vi "Autonomous Independent.vi"   [LabVIEW 2013]
doc: "This VI is called when autonomous begins, and will automatically be terminated when autonomous ends. You can carry out timed or sensor driven robot movement independently without needing to return to the caller."
uses:
  Robot Global Data.vi
  <vilib>/Rock Robotics/WPI/Counter/WPI_CounterDigitalInputToDigitalSource.vi
types:
  T1 = cluster{"Open Claw?":bool, "Close Claw?":bool, "Minibot Out":bool}
  T2 = typedef "WPI_DigitalInputDevRef.ctl" = cluster{"DevStatus":errorcluster, "DIO Channel":T3, "Digital Module":T4}
  T3 = typedef "FPGA_DIOChannel.ctl" = enum8{"DIO 1", "DIO 2", "DIO 3", "DIO 4", "DIO 5", "DIO 6", "DIO 7", "DIO 8", "DIO 9", "DIO 10", "DIO 11", "DIO 12", "DIO 13", "DIO 14", "Invalid"}
  T4 = typedef "FPGA_TypedefDigitalModule.ctl" = enum16{"Digital Module 1", "Digital Module 2"}
  T5 = typedef "FPGA_CounterEncoderSourceConvertionLVSourceType.ctl" = cluster{"DevStatus":errorcluster, "AnalogTriggerMode?":bool, "DigitalMode":cluster{"Digital Module":T4, "DIO Channel":T6}, "AnalogTriggerMode":cluster{"AnalogTriggerIndex":T7, "OutputType":T8}}
  T6 = typedef "FPGA_DIODigitalSourceChannel.ctl" = enum8{"DIO 1", "DIO 2", "DIO 3", "DIO 4", "DIO 5", "DIO 6", "DIO 7", "DIO 8", "DIO 9", "DIO 10", "DIO 11", "DIO 12", "DIO 13", "DIO 14", "Disabled"}
  T7 = typedef "FPGA_AnalogTriggerIndex.ctl" = enum8{"Trig 0", "Trig 1", "Trig 2", "Trig 3", "Trig 4", "Trig 5", "Trig 6", "Trig 7", "Invalid"}
  T8 = typedef "FPGA_AnalogTriggerOutType.ctl" = enum16{"InWindow", "TriggerState", "Rising", "Falling"}
  T9 = typedef "WPI_InterruptRef.ctl" = cluster{"DevStatus":errorcluster, "InterruptIndex":T10}
  T10 = typedef "FPGA_InterruptIndex.ctl" = enum8{"0", "1", "2", "3", "4", "5", "6", "7", "Invalid"}
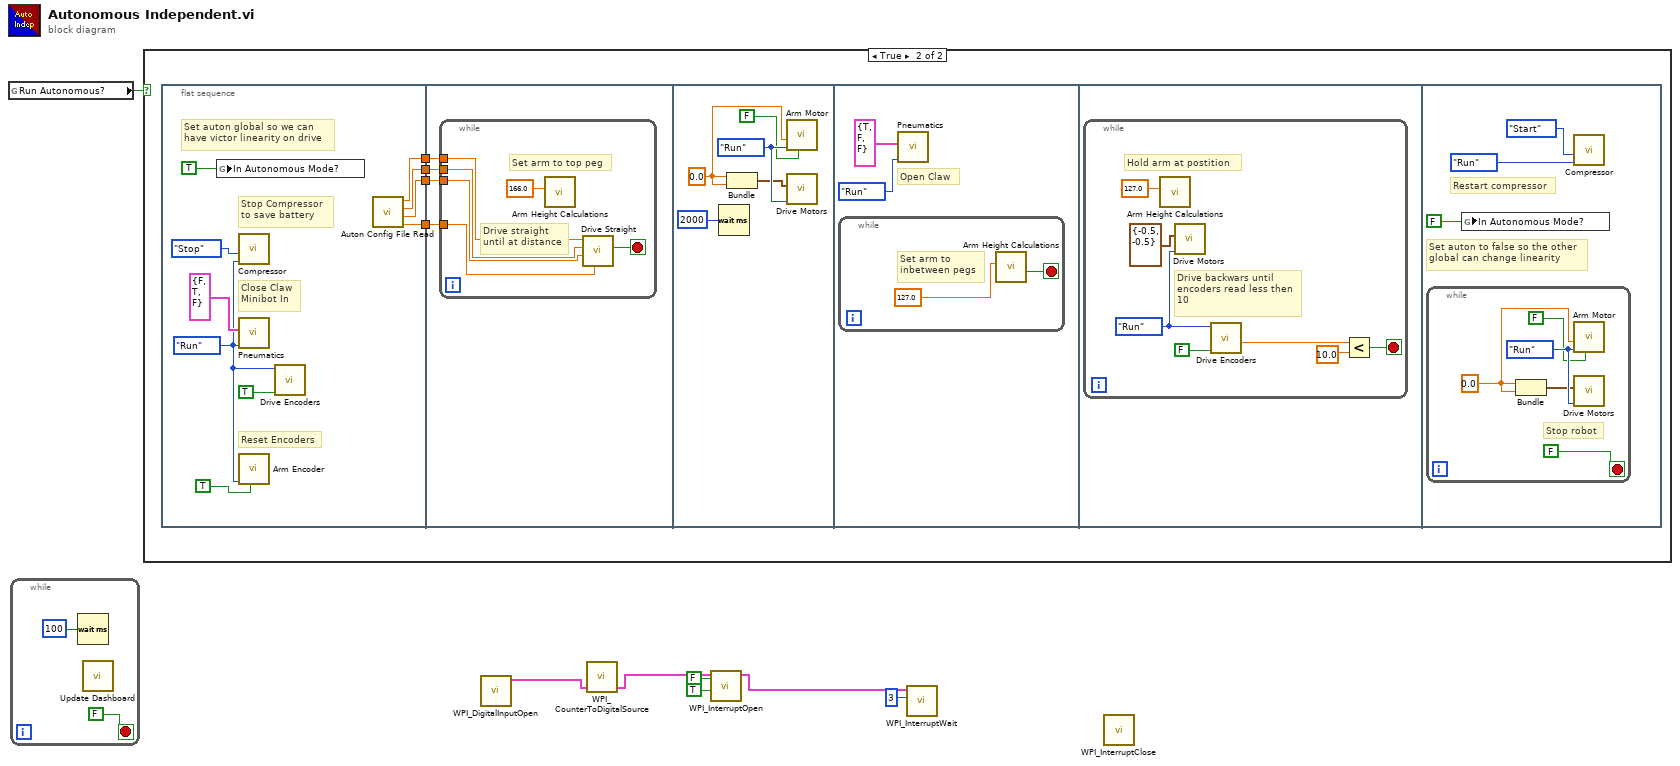
[diagram p0: block diagram]
diagram:
  n1 = global read "Robot Global Data.vi" "Run Autonomous?"() -> (w7:bool)
  n2 = while {
    stop <- FALSE stop-if-true
    n3 = Wait (ms)(milliseconds to wait=u32 100) -> ()  [unwired: 1 out]
    n4 = call "Update Dashboard.vi"() -> ()  [unwired: 12 out]
  }
  n5 = case shown="True" w7 {
    frame False {
    }
    frame True {
      n6 = flat-sequence {
        tunnel: [w17] -> w13
        tunnel: [w16] -> w12
        tunnel: [w15] -> w11
        tunnel: [w14] -> w10
        tunnel: w13 -> [w27]
        tunnel: w12 -> [w26]
        tunnel: w11 -> [w25]
        tunnel: w10 -> [w24]
        frame #0 {
          w19 = enum16{"Init", "Run", "End"}."Run" ("Mode")
          # "Set auton global so we can\nhave victor linearity on drive"
          # "Stop Compressor\nto save battery"
          # "Close Claw\nMinibot In"
          # "Reset Encoders"
          n7 = global write "Robot Global Data.vi" "In Autonomous Mode?"(TRUE ("In Autonomous Mode?")) -> ()
          n8 = call "Compressor.vi"("Mode"=w19, "Compressor State"=enum32{"Start", "Stop"}."Stop") -> ()  [unwired: 2 in, 8 out]
          n9 = call "Pneumatics.vi"("Mode"=w19, "Inputs"=T1 {"Open Claw?"=FALSE, "Close Claw?"=TRUE, "Minibot Out"=FALSE}) -> ()  [unwired: 1 in, 9 out]
          n10 = call "Arm Encoder.vi"("Reset Encoder?"=TRUE, "Mode"=w19) -> ()  [unwired: 1 in, 9 out]
          n11 = call "Drive Encoders.vi"("Reset Encoders?"=TRUE, "Mode"=w19) -> ()  [unwired: 2 in, 8 out]
          n12 = call "Auton Config File Read.vi"() -> ("GainSlow"=w14:dbl, "Distance"=w16:dbl, "Speed"=w15:dbl, "GainFast"=w17:dbl)
        }
        frame #1 {
          n13 = while {
            tunnel: w27 -> [w31]
            tunnel: w26 -> [w30]
            tunnel: w25 -> [w29]
            tunnel: w24 -> [w28]
            stop <- w32 stop-if-true
            # "Drive straight\nuntil at distance"
            # "Set arm to top peg"
            n14 = call "Arm Height Calculations.vi"("Height Input"=166.0) -> ()  [unwired: 11 out]
            n15 = call "Drive Straight.vi"("Encoder Gain - Slow"=w28, "Distance"=w30, "Speed"=w29, "Encoder Gain - Fast"=w31) -> ("At Distance"=w32:bool)  [unwired: 7 out]
          }
        }
        frame #2 {
          w36 = 0.0
          w38 = enum16{"Init", "Run", "End"}."Run" ("Mode")
          n16 = Wait (ms)(milliseconds to wait=u32 2000) -> ()  [unwired: 1 out]
          n17 = Bundle(w36, w36) -> (w35:cluster{dbl, dbl})  [unwired: 1 out]
          n18 = call "Arm Motor.vi"("Stall Arm?"=FALSE, "Mode"=w38, "Arm motor speed"=w36) -> ()  [unwired: 1 in, 8 out]
          n19 = call "Drive Motors.vi"("Mode"=w38, "Inputs"=w35) -> ()  [unwired: 1 in, 9 out]
        }
        frame #3 {
          # "Open Claw"
          n20 = while {
            stop <- w41 stop-if-true
            # "Set arm to\ninbetween pegs"
            n21 = call "Arm Height Calculations.vi"("Height Input"=127.0) -> ("At Height?"=w41:bool)  [unwired: 10 out]
          }
          n22 = call "Pneumatics.vi"("Mode"=enum16{"Init", "Run", "End"}."Run", "Inputs"=T1 {"Open Claw?"=TRUE, "Close Claw?"=FALSE, "Minibot Out"=FALSE}) -> ()  [unwired: 1 in, 9 out]
        }
        frame #4 {
          n23 = while {
            stop <- w44 stop-if-true
            w48 = enum16{"Init", "Run", "End"}."Run" ("Mode")
            # "Drive backwars until\nencoders read less then\n10"
            # "Hold arm at postition"
            n24 = call "Arm Height Calculations.vi"("Height Input"=127.0) -> ()  [unwired: 11 out]
            n25 = call "Drive Motors.vi"("Mode"=w48, "Inputs"=cluster{"Left Drive":dbl, "Right Drive":dbl} {"Left Drive"=-0.5, "Right Drive"=-0.5}) -> ()  [unwired: 1 in, 9 out]
            n26 = call "Drive Encoders.vi"("Reset Encoders?"=FALSE, "Mode"=w48) -> ("Average Distance"=w46:dbl)  [unwired: 2 in, 7 out]
            n27 = Less?(x=w46, y=10.0) -> (x < y?=w44:bool)
          }
        }
        frame #5 {
          # "Set auton to false so the other\nglobal can change linearity"
          # "Restart compressor"
          n28 = while {
            stop <- FALSE stop-if-true
            w55 = 0.0
            w57 = enum16{"Init", "Run", "End"}."Run" ("Mode")
            # "Stop robot"
            n29 = Bundle(w55, w55) -> (w54:cluster{dbl, dbl})  [unwired: 1 out]
            n30 = call "Arm Motor.vi"("Stall Arm?"=FALSE, "Mode"=w57, "Arm motor speed"=w55) -> ()  [unwired: 1 in, 8 out]
            n31 = call "Drive Motors.vi"("Mode"=w57, "Inputs"=w54) -> ()  [unwired: 1 in, 9 out]
          }
          n32 = global write "Robot Global Data.vi" "In Autonomous Mode?"(FALSE ("In Autonomous Mode?")) -> ()
          n33 = call "Compressor.vi"("Mode"=enum16{"Init", "Run", "End"}."Run", "Compressor State"=enum32{"Start", "Stop"}."Start") -> ()  [unwired: 2 in, 8 out]
        }
      }
    }
  }
  n34 = call <vilib>:"WPI_DigitalInputOpen.vi"() -> ("DigitalInputDevRef"=w6:T2)  [unwired: 10 in, 1 out]
  n35 = call-poly <vilib>:"WPI_CounterToDigitalSource.vi"("DigitalInputDevRef"=w6) -> ("Digital Source"=w5:T5)  [unwired: 6 in]
  n36 = call <vilib>:"WPI_InterruptOpen.vi"("Falling Edge"=TRUE, "Rising Edge"=FALSE, "Source"=w5) -> ("InterruptRef"=w2:T9)  [unwired: 7 in, 1 out]
  n37 = call <vilib>:"WPI_InterruptWait.vi"("Timeout (ms)"=3, "InterruptRef"=w2) -> ()  [unwired: 6 in, 4 out]
  n38 = call <vilib>:"WPI_InterruptClose.vi"() -> ()  [unwired: 11 in, 1 out]
